vi "AlliGator Add Python Functions to Object Menu.vi"(8 "error in (no error)":errorcluster, 10 "Menu in":refnum<k9>, 11 "Object Refnum":refnum<vi>) -> (0 "error out":errorcluster, 2 "Menu out":refnum<k9>, 3 "Object Refnum dup":refnum<vi>)   [LabVIEW 2021, in "AlliGator Python Plugins.lvlib"]
doc: "Adds python function to object menu."
uses:
  AlliGator Python Plugins.lvlib
panel:
  # "see the AlliGator License on the block diagram (Ctrl+E or Window:Show Block Diagram)"
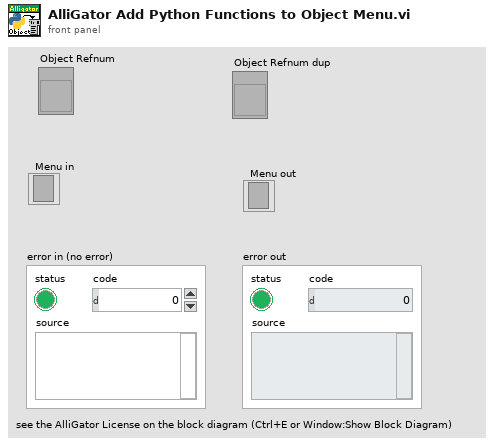
[diagram p1: front panel]
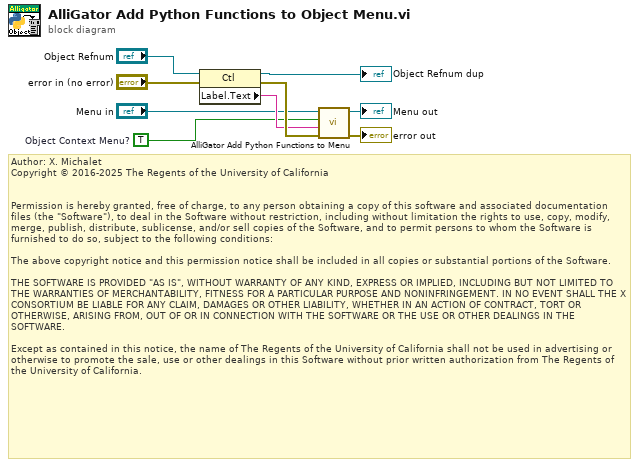
[diagram p0: block diagram]
diagram:
  w1 = TRUE  # Object Context Menu?
  # "Author: X. Michalet\nCopyright © 2016-2025 The Regents of the University of California\n \n\nPermission is hereby granted, free of charge, to any person obtaining a copy of this software and associated documentation files (the \"Software\"), to deal in the Software without restriction, including without limitation the rights to use, copy, modify, merge, publish, distribute, sublicense, and/or sell copies of the Software, and to permit persons to whom the Software is furnished to do so, subject to the following conditions:\n\nThe above copyright notice and this permission notice shall be included in all copies or substantial portions of the Software.\n\nTHE SOFTWARE IS PROVIDED \"AS IS\", WITHOUT WARRANTY OF ANY KIND, EXPRESS OR IMPLIED, INCLUDING BUT NOT LIMITED TO THE WARRANTIES OF MERCHANTABILITY, FITNESS FOR A PARTICULAR PURPOSE AND NONINFRINGEMENT. IN NO EVENT SHALL THE X CONSORTIUM BE LIABLE FOR ANY CLAIM, DAMAGES OR OTHER LIABILITY, WHETHER IN AN ACTION OF CONTRACT, TORT OR OTHERWISE, ARISING FROM, OUT OF OR IN CONNECTION WITH THE SOFTWARE OR THE USE OR OTHER DEALINGS IN THE SOFTWARE.\n\nExcept as contained in this notice, the name of The Regents of the University of California shall not be used in advertising or otherwise to promote the sale, use or other dealings in this Software without prior written authorization from The Regents of the University of California."
  n1 = property class="Ctl"(reference="Object Refnum", error in="error in (no error)") -> (reference out=→"Object Refnum dup":refnum<vi>, error out=w9:errorcluster, "Label.Text"=w7:string)
  n2 = call "AlliGator Add Python Functions to Menu.vi"("error in (no error)"=w9, "Parent Menu Tag"=w7, "Object Context Menu?"=w1, "Menu in"="Menu in") -> ("error out"=→"error out":errorcluster, "Menu out"=→"Menu out":refnum<k9>)  [unwired: 6 in]
